vi "KNRmOS6Delta put obiect.vi"(7 "move to":T1(ring), 8 "error in (no error)":errorcluster, 10 "off setY":dbl, 11 "off setX":dbl=10.0) -> (0 "error in (no error) 2":errorcluster)   [LabVIEW 2019]
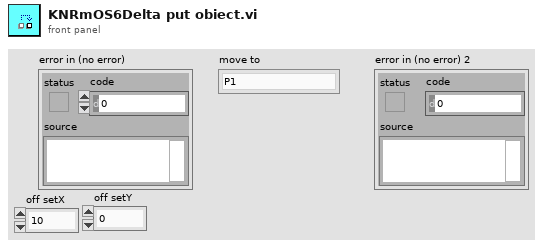
[diagram p1: front panel]
types:
  T1 = enum16{"P1", "P2", "P3", "P4", "P5", "P6", "OUT", "take a picture"}
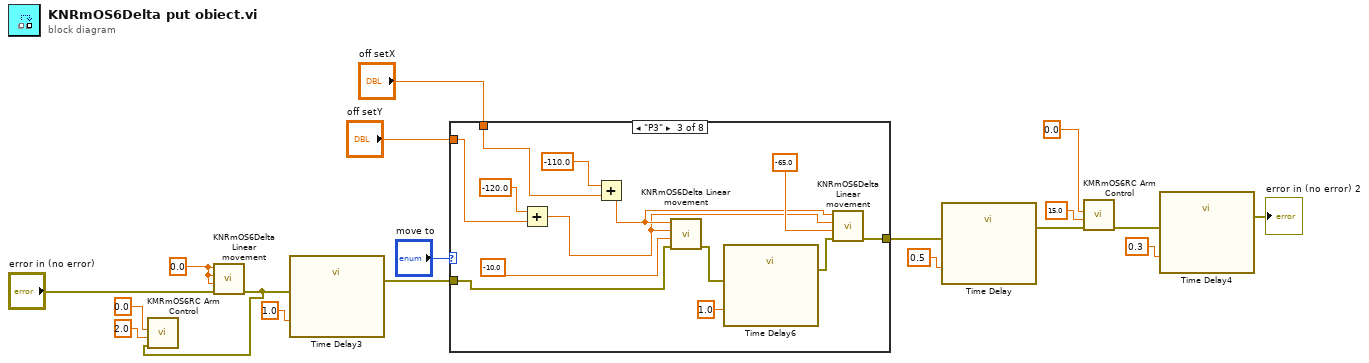
[diagram p0: block diagram]
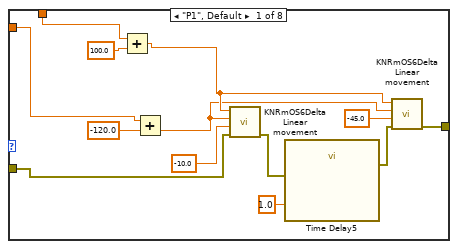
[diagram p2: hidden frame]
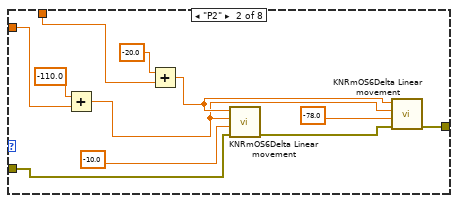
[diagram p3: hidden frame]
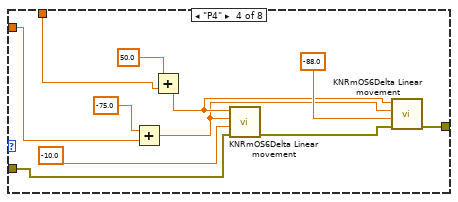
[diagram p4: hidden frame]
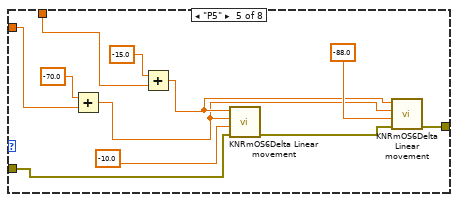
[diagram p5: hidden frame]
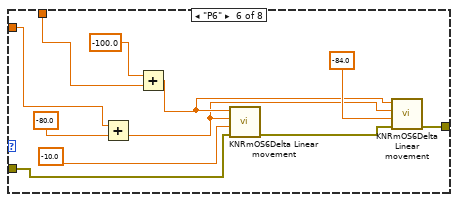
[diagram p6: hidden frame]
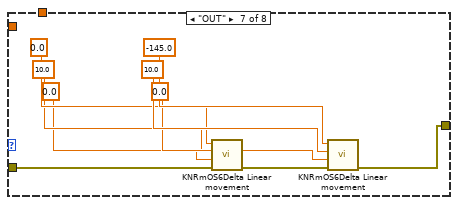
[diagram p7: hidden frame]
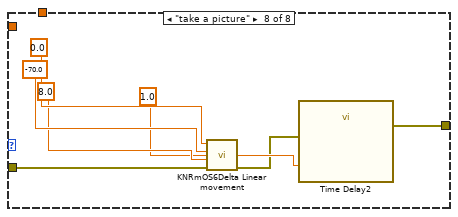
[diagram p8: hidden frame]
diagram:
  w18 = 0.0 ("x0")
  n1 = call "KNRmOS6Delta Linear movement.vi"("error in (no error)"="error in (no error)", "z0"=w18, "y0"=w18, "x0"=w18) -> ("error out"=w3:errorcluster)  [unwired: 7 in]
  n2 = call "KMRmOS6RC Arm Control.vi"("error in (no error)"=w3, "clip"=2.0, "turn"=0.0) -> ()  [unwired: 6 in, 3 out]
  n3 = call "Time Delay3"("error in (no error)"=w3, "Delay Time (s)"=1.0 ("x0")) -> ("error out"=w8:errorcluster)  [unwired: 9 in]
  n4 = case shown="\"P3\"" "move to" {
    tunnel: w8 -> [w29 w40 w53 w64 w75 w86 w93 w101]
    tunnel: [w31 w41 w54 w65 w76 w87 w94 w98] -> w12
    tunnel: "off setX" -> [w24 w34 w48 w58 w69 w80 _ _]
    tunnel: "off setY" -> [w22 w32 w46 w56 w67 w78 _ _]
    frame "P1", Default {
      n5 = Add(x=w24, y=100.0 ("x0")) -> (x+y=w25:dbl)
      n6 = Add(x=w22, y=-120.0 ("y0")) -> (x+y=w23:dbl)
      n7 = call "KNRmOS6Delta Linear movement.vi"("error in (no error)"=w29, "z0"=-10.0, "y0"=w23, "x0"=w25) -> ("error out"=w20:errorcluster)  [unwired: 7 in]
      n8 = call "Time Delay5"("error in (no error)"=w20, "Delay Time (s)"=1.0) -> ("error out"=w19:errorcluster)  [unwired: 9 in]
      n9 = call "KNRmOS6Delta Linear movement.vi"("error in (no error)"=w19, "z0"=-45.0, "y0"=w23, "x0"=w25) -> ("error out"=w31:errorcluster)  [unwired: 7 in]
    }
    frame "P2" {
      n10 = Add(x=-110.0 ("y0"), y=w32) -> (x+y=w33:dbl)
      n11 = Add(x=-20.0 ("x0"), y=w34) -> (x+y=w35:dbl)
      n12 = call "KNRmOS6Delta Linear movement.vi"("error in (no error)"=w40, "z0"=-10.0, "y0"=w33, "x0"=w35) -> ("error out"=w39:errorcluster)  [unwired: 7 in]
      n13 = call "KNRmOS6Delta Linear movement.vi"("error in (no error)"=w39, "z0"=-78.0, "y0"=w33, "x0"=w35) -> ("error out"=w41:errorcluster)  [unwired: 7 in]
    }
    frame "P3" {
      n14 = Add(x=-120.0 ("y0"), y=w46) -> (x+y=w47:dbl)
      n15 = Add(x=-110.0 ("x0"), y=w48) -> (x+y=w49:dbl)
      n16 = call "KNRmOS6Delta Linear movement.vi"("error in (no error)"=w53, "z0"=-10.0, "y0"=w47, "x0"=w49) -> ("error out"=w44:errorcluster)  [unwired: 7 in]
      n17 = call "Time Delay6"("error in (no error)"=w44, "Delay Time (s)"=1.0) -> ("error out"=w43:errorcluster)  [unwired: 9 in]
      n18 = call "KNRmOS6Delta Linear movement.vi"("error in (no error)"=w43, "z0"=-65.0, "y0"=w47, "x0"=w49) -> ("error out"=w54:errorcluster)  [unwired: 7 in]
    }
    frame "P4" {
      n19 = Add(x=-75.0 ("y0"), y=w56) -> (x+y=w57:dbl)
      n20 = Add(x=50.0 ("x0"), y=w58) -> (x+y=w59:dbl)
      n21 = call "KNRmOS6Delta Linear movement.vi"("error in (no error)"=w64, "z0"=-10.0, "y0"=w57, "x0"=w59) -> ("error out"=w63:errorcluster)  [unwired: 7 in]
      n22 = call "KNRmOS6Delta Linear movement.vi"("error in (no error)"=w63, "z0"=-88.0, "y0"=w57, "x0"=w59) -> ("error out"=w65:errorcluster)  [unwired: 7 in]
    }
    frame "P5" {
      n23 = Add(x=-70.0 ("y0"), y=w67) -> (x+y=w68:dbl)
      n24 = Add(x=-15.0 ("x0"), y=w69) -> (x+y=w70:dbl)
      n25 = call "KNRmOS6Delta Linear movement.vi"("error in (no error)"=w75, "z0"=-10.0, "y0"=w68, "x0"=w70) -> ("error out"=w74:errorcluster)  [unwired: 7 in]
      n26 = call "KNRmOS6Delta Linear movement.vi"("error in (no error)"=w74, "z0"=-88.0, "y0"=w68, "x0"=w70) -> ("error out"=w76:errorcluster)  [unwired: 7 in]
    }
    frame "P6" {
      n27 = Add(x=w78, y=-80.0 ("y0")) -> (x+y=w79:dbl)
      n28 = Add(x=-100.0 ("x0"), y=w80) -> (x+y=w81:dbl)
      n29 = call "KNRmOS6Delta Linear movement.vi"("error in (no error)"=w86, "z0"=-10.0, "y0"=w79, "x0"=w81) -> ("error out"=w85:errorcluster)  [unwired: 7 in]
      n30 = call "KNRmOS6Delta Linear movement.vi"("error in (no error)"=w85, "z0"=-84.0, "y0"=w79, "x0"=w81) -> ("error out"=w87:errorcluster)  [unwired: 7 in]
    }
    frame "OUT" {
      n31 = call "KNRmOS6Delta Linear movement.vi"("error in (no error)"=w93, "z0"=0.0, "y0"=10.0, "x0"=0.0) -> ("error out"=w92:errorcluster)  [unwired: 7 in]
      n32 = call "KNRmOS6Delta Linear movement.vi"("error in (no error)"=w92, "z0"=0.0, "y0"=10.0, "x0"=-145.0) -> ("error out"=w94:errorcluster)  [unwired: 7 in]
    }
    frame "take a picture" {
      n33 = call "KNRmOS6Delta Linear movement.vi"("error in (no error)"=w101, "z0"=8.0, "y0"=-70.0, "x0"=0.0) -> ("error out"=w99:errorcluster)  [unwired: 7 in]
      n34 = call "Time Delay2"("error in (no error)"=w99, "Delay Time (s)"=1.0) -> ("error out"=w98:errorcluster)  [unwired: 9 in]
    }
  }
  n35 = call "Time Delay"("error in (no error)"=w12, "Delay Time (s)"=0.5) -> ("error out"=w11:errorcluster)  [unwired: 9 in]
  n36 = call "KMRmOS6RC Arm Control.vi"("error in (no error)"=w11, "clip"=15.0, "turn"=0.0) -> ("error out"=w6:errorcluster)  [unwired: 6 in, 2 out]
  n37 = call "Time Delay4"("error in (no error)"=w6, "Delay Time (s)"=0.3) -> ("error out"=→"error in (no error) 2":errorcluster)  [unwired: 9 in]
